vi "Der_Sigmoid.vi"(1 "A_l":T1) -> (0 "g'(Z)":T1)   [LabVIEW 2016]
uses:
  <vilib>/Analysis/Matrix/Datatypes/RealMatrix.ctl
  <vilib>/Analysis/Matrix/Numeric/Conversions/Matrix To Array - RM.vi
  <vilib>/Analysis/Matrix/Numeric/Conversions/Array To Matrix - RA2.vi
  <vilib>/Analysis/Matrix/NI_Matrix.lvlib
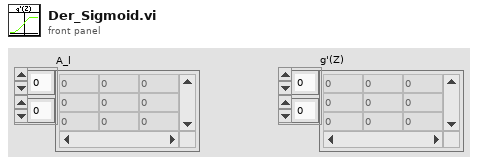
[diagram p1: front panel]
types:
  T1 = typedef "NI_Matrix.lvlib/RealMatrix.ctl" = dbl[][]
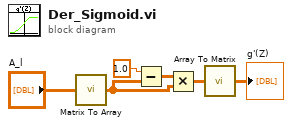
[diagram p0: block diagram]
diagram:
  n1 = call-poly <vilib>:"Matrix To Array.vi"("Real Matrix"="A_l") -> ("Real 2D Array"=w3:dbl[][])
  n2 = Subtract ("Subtract.vi")(x=1.0, y=w3) -> (x-y=w4:dbl[][])
  n3 = Multiply(x=w4, y=w3) -> (x*y=w2:dbl[][])
  n4 = call-poly <vilib>:"Array To Matrix.vi"("Real 2D Array"=w2) -> ("Real Matrix"=→"g'(Z)":T1)
